vi "PLCtoGUIBool.vi"(9 "SubOffset":u16, 10 "DB Input Vals":u8[](array[numeric])=[0, 0, 0, 0]) -> (2 "element":bool)   [LabVIEW 2023]
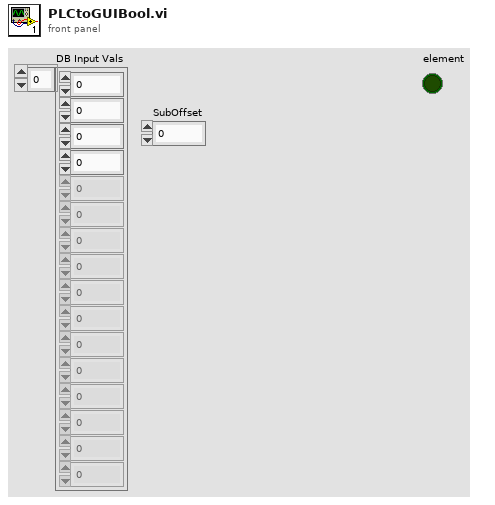
[diagram p1: front panel]
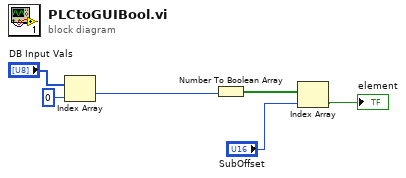
[diagram p0: block diagram]
diagram:
  n1 = Index Array(array="DB Input Vals", index=0) -> (element=w6:u8)
  n2 = Number To Boolean Array(number=w6) -> (Boolean array=w3:bool[])
  n3 = Index Array(array=w3, index="SubOffset") -> (element=→"element":bool)
